vi "Compile Current Sense.vi"(8 "error in (no error)":errorcluster, 11 "Device Item Ref in":T5 format="%.0x") -> (0 "error out":errorcluster, 1 "Wheel Speed Sensor Engine Data":T1 {"Ordered Channels" format="%.0x"; "RT IDs"."Slot #" max=15; "RT IDs"."Chip Address (A2 A1 A0)" max=7}, 2 "Initial Wheel Speed Sensor SPI CMDs":u64[](array[numeric]), 3 "Device Item Ref out":T5 format="%.0x")   [LabVIEW 2014, in "SLSC configuration System Explorer.lvlib"]
uses:
  <vilib>/NI Veristand/Custom Device API/Custom Device Item Ref.ctl
  Shared/Type Defs/RT Engine Data.ctl
  Shared/Type Defs/RT IDs.ctl
  Shared/SPI Utility/Slot #.ctl
  Shared/MCP23S17/Chip Address.ctl
  Shared/Constants.vi
  SLSC configuration System Explorer.lvlib
  <vilib>/NI Veristand/Custom Device Tools/Custom Device Utility Library/Custom Device Utility Library.lvlib
  Shared/SLSC configuration Shared.lvlib
  <vilib>/NI Veristand/Custom Device API/Custom Device API.lvlib
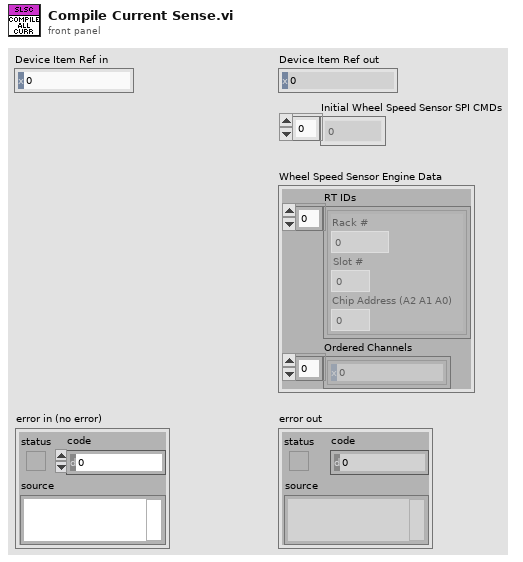
[diagram p1: front panel]
types:
  T1 = typedef "SLSC configuration Shared.lvlib/RT Engine Data.ctl" = cluster{"RT IDs":T2[], "Ordered Channels":T5[]}
  T2 = typedef "SLSC configuration Shared.lvlib/RT IDs.ctl" = cluster{"Rack #":u8, "Slot #":T3, "Chip Address (A2 A1 A0)":T4}
  T3 = typedef "SLSC configuration Shared.lvlib/Slot #.ctl" = u8
  T4 = typedef "SLSC configuration Shared.lvlib/Chip Address.ctl" = u8
  T5 = typedef "Custom Device API.lvlib/Custom Device Item Ref.ctl" = u64
  T6 = typedef "SLSC configuration Shared.lvlib/Card Position.ctl" = cluster{"Rack #":u8, "Slot #":T3}
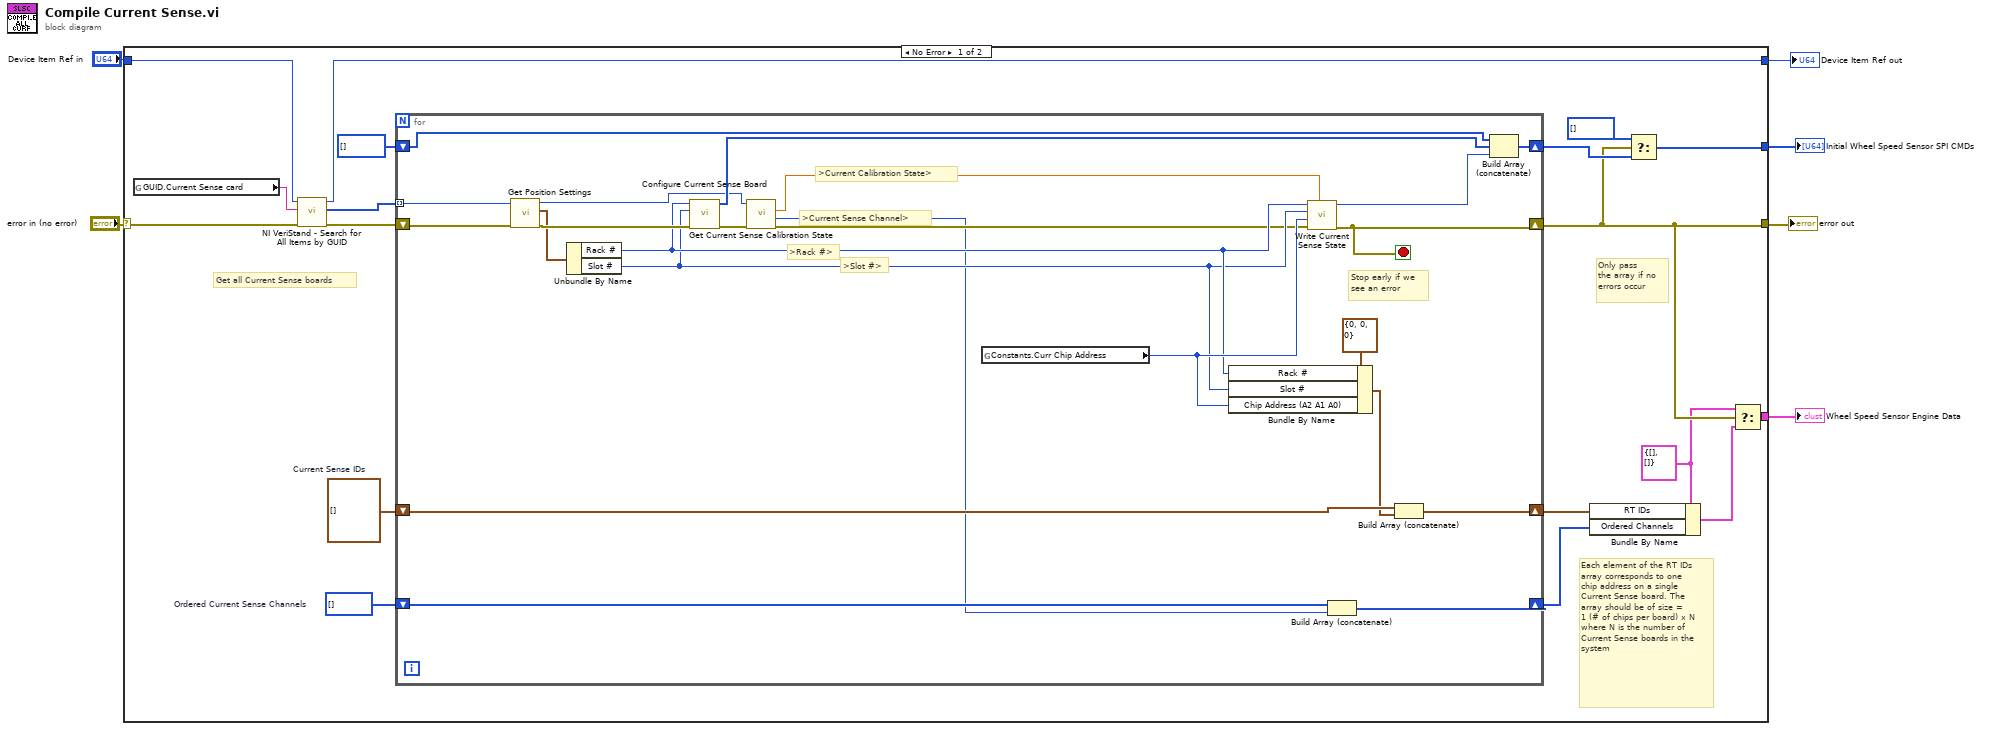
[diagram p0: block diagram]
diagram:
  n1 = case shown="No Error" "error in (no error)" {
    selector: "error in (no error)" -> [w21 w49]
    tunnel: [w10 w49] -> w6
    tunnel: "Device Item Ref in" -> [w15 w48]
    tunnel: [w7 _] -> w3
    tunnel: [w11 _] -> w2
    tunnel: [w14 w48] -> w1
    frame No Error {
      w9 = T1 {"RT IDs"=[], "Ordered Channels"=[]} ("FIU Engine Data")
      w18 = T5[] []  # Ordered Current Sense Channels
      w19 = T2[] []  # Current Sense IDs
      # "Only pass\nthe array if no\nerrors occur"
      # "Get all Current Sense boards"
      # "Each element of the RT IDs array corresponds to one chip address on a single Current Sense board. The array should be of size =\n1 (# of chips per board) x N where N is the number of Current Sense boards in the system"
      n2 = global read "Constants.vi" "GUID.Current Sense card"() -> (w24:string)
      n3 = call <vilib>:"NI VeriStand - Search for All Items by GUID.vi"("error in"=w21, "Item GUID"=w24, "Section Ref in"=w15) -> ("error out"=w23:errorcluster, "Item Refs"=w22:T5[], "Section Ref out"=w14:T5)  [unwired: 5 in, 1 out]
      n4 = for {
        tunnel: w22 -> [w35] mode=indexing
        shift-right: [w39] -> w10
        shift-left: w23 -> [w34]
        shift-right: [w44] -> w13
        shift-left: u64[] [] ("SPI FIFO Messages") -> [w47]
        shift-right: [w42] -> w17
        shift-left: w19 -> [w43]
        shift-right: [w40] -> w16
        shift-left: w18 -> [w41]
        stop <- w39 stop-if-true
        # ">Current Calibration State>"
        # "Stop early if we\nsee an error"
        # ">Current Sense Channel>"
        # ">Slot #>"
        # ">Rack #>"
        n5 = call "Get Position Settings.vi"("error in (no error)"=w34, "Item Ref in"=w35) -> ("error out"=w33:errorcluster, "Card Position"=w32:T6, "Item Ref out"=w28:T5)  [unwired: 7 in]
        n6 = Unbundle By Name(w32) -> ("Rack #"=w31:u8, "Slot #"=w30:T3)
        n7 = call "Configure Current Sense Board.vi"("error in (no error)"=w33, "Slot #"=w30, "Rack #"=w31) -> ("error out"=w29:errorcluster, "SPI FIFO Messages"=w46:u64[])  [unwired: 7 in]
        n8 = call "Get Current Sense Calibration State.vi"("error in (no error)"=w29, "Item Ref in"=w28) -> ("error out"=w27:errorcluster, "Current Sense Channel"=w26:T5, "Calibration State"=w25:dbl)  [unwired: 6 in, 1 out]
        n9 = global read "Constants.vi" "Constants.Curr Chip Address"() -> (w38:u8)
        n10 = Bundle By Name(cluster=T2 {"Rack #"=0, "Slot #"=0, "Chip Address (A2 A1 A0)"=0}, "Rack #"=w31, "Slot #"=w30, "Chip Address (A2 A1 A0)"=w38) -> (w36:T2)
        n11 = call "Write Current Sense State.vi"("Current Sense Calibration State"=w25, "error in (no error)"=w27, "Chip Address (A2 A1 A0)"=w38, "Slot #"=w30, "Rack #"=w31) -> ("error out"=w39:errorcluster, "FIFO SPI Message"=w45:u64)  [unwired: 4 in, 1 out]
        n12 = Build Array (concatenate)(w41, w26) -> (w40:T5[])
        n13 = Build Array (concatenate)(w43, w36) -> (w42:T2[])
        n14 = Build Array (concatenate)(w47, w46, w45) -> (w44:u64[])
      }
      n15 = Bundle By Name(cluster=w9, "RT IDs"=w17, "Ordered Channels"=w16) -> (w8:T1)
      n16 = Select(t=u64[] [], s=w10, f=w13) -> (s? t:f=w11:u64[])
      n17 = Select(t=w9, s=w10, f=w8) -> (s? t:f=w7:T1)
    }
    frame Error {
    }
  }
  "error out" <- w6
  "Device Item Ref out" <- w1
  "Wheel Speed Sensor Engine Data" <- w3
  "Initial Wheel Speed Sensor SPI CMDs" <- w2
